vi "CylSet.vi"(4 "Cycle off":dbl[unit], 6 "Cycle on":dbl[unit], 8 "error in (no error)":errorcluster, 9 "Tag":string, 10 "SEQ Pool":T1(array[cluster]) {"Delay Time" format="%.3f"}, 11 "Cycle in":refnum<class "Cycle.lvclass">) -> (0 "error out":errorcluster, 3 "Cycle out":refnum<class "Cycle.lvclass">)   [LabVIEW 2012, in "Cycle.lvclass"]
uses:
  Cycle.lvclass
  Sequence.lvclass
  Cycle.lvclass/Cycle.ctl
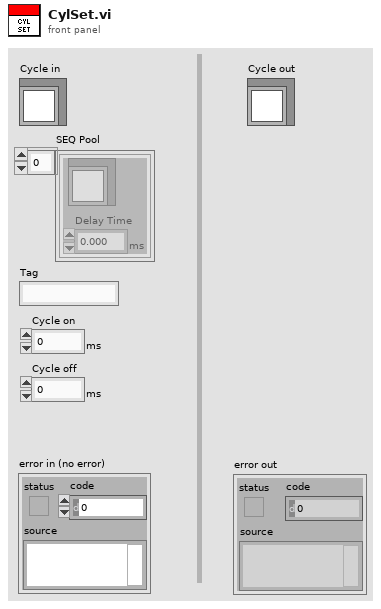
[diagram p1: front panel]
types:
  T1 = cluster{"Sequence.lvclass":refnum<class "Sequence.lvclass">, "Delay Time":dbl[unit]}[]
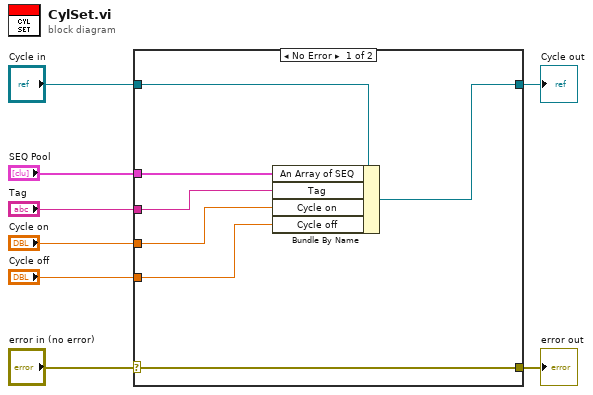
[diagram p0: block diagram]
diagram:
  n1 = case shown="No Error" "error in (no error)" {
    selector: "error in (no error)" -> [w15 w16]
    tunnel: [w15 w16] -> w7
    tunnel: [w13 w17] -> w5
    tunnel: "Cycle in" -> [w14 w17]
    tunnel: "SEQ Pool" -> [w9 _]
    tunnel: "Tag" -> [w12 _]
    tunnel: "Cycle on" -> [w11 _]
    tunnel: "Cycle off" -> [w10 _]
    frame No Error {
      n2 = Bundle By Name(cluster=w14, "An Array of SEQ"=w9, "Tag"=w12, "Cycle on"=w11, "Cycle off"=w10) -> (w13:refnum<class "Cycle.lvclass">)
    }
    frame Error {
    }
  }
  "error out" <- w7
  "Cycle out" <- w5
